vi "Load_Breast_Cancer.vi"(8 "error in":errorcluster caption="entrée d'erreur") -> (0 "error out":errorcluster caption="sortie d'erreur", 3 "Tableau":string[][](array[string]))   [LabVIEW 2020]
doc: "Data Set Characteristics :\n\nNumber of Instances : 569\n\nNumber of Attributes : 30 numeric, predictive attributes and the class\n\nAttribute Information : \n - radius (mean of distances from center to points on the perimeter)\n - texture (standard deviation of gray-scale values)\n - perimeter\n - area\n - smoothness (local variation in radius lengths)\n - compactness (perimeter^2 / area - 1.0)\n - concavity (severity of concave portions of the contour)\n - concave points (number of concave portions of the contour)\n - symmetry\n - fractal dimension (“coastline approximation” - 1)\n\nThe mean, standard error, and “worst” or largest (mean of the three worst/largest values) of these features were computed for each image, resulting in 30 features. For instance, field 0 is Mean Radius, field 10 is Radius SE, field 20 is Worst Radius.\n\nclass :\n - WDBC-Malignant\n - WDBC-Benign\n\nSummary Statistics : \n\n - radius (mean) : 6.981 28.11\n - texture (mean) : 9.71 39.28\n - perimeter (mean) : 43.79 188.5\n - area (mean) : 143.5 2501.0\n - smoothness (mean) : 0.053 0.163\n - compactness (mean) : 0.019 0.345\n - concavity (mean) : 0.0 0.427\n - concave points (mean) : 0.0 0.201\n - symmetry (mean) : 0.106 0.304\n - fractal dimension (mean) : 0.05 0.097\n - radius (standard error) : 0.112 2.873\n - texture (standard error) : 0.36 4.885\n - perimeter (standard error) : 0.757 21.98\n - area (standard error) : 6.802 542.2\n - smoothness (standard error) : 0.002 0.031\n - compactness (standard error) : 0.002 0.135\n - concavity (standard error) : 0.0 0.396\n - concave points (standard error) : 0.0 0.053\n - symmetry (standard error) : 0.008 0.079\n - fractal dimension (standard error): 0.001 0.03\n - radius (worst) : 7.93 36.04\n - texture (worst) : 12.02 49.54\n - perimeter (worst) : 50.41 251.2\n - area (worst) : 185.2 4254.0\n - smoothness (worst) : 0.071 0.223\n - compactness (worst) : 0.027 1.058\n - concavity (worst) : 0.0 1.252\n - concave points (worst) : 0.0 0.291\n - symmetry (worst) : 0.156 0.664\n - fractal dimension (worst) : 0.055 0.208\n\nMissing Attribute Values : None\n\nClass Distribution : \n - 212 - Malignant \n - 357 - Benign\n\nCreator : Dr. William H. Wolberg, W. Nick Street, Olvi L. Mangasarian\n\nDonor : Nick Street\n\nDate : November, 1995\n\nThis is a copy of UCI ML Breast Cancer Wisconsin (Diagnostic) datasets. https://goo.gl/U2Uwz2\n\nFeatures are computed from a digitized image of a fine needle aspirate (FNA) of a breast mass. They describe characteristics of the cell nuclei present in the image.\n\nSeparating plane described above was obtained using Multisurface Method-Tree (MSM-T) [K. P. Bennett, “Decision Tree Construction Via Linear Programming.” Proceedings of the 4th Midwest Artificial Intelligence and Cognitive Science Society, pp. 97-101, 1992], a classification method which uses linear programming to construct a decision tree. Relevant features were selected using an exhaustive search in the space of 1-4 features and 1-3 separating planes.\n\nThe actual linear program used to obtain the separating plane in the 3-dimensional space is that described in: [K. P. Bennett and O. L. Mangasarian: “Robust Linear Programming Discrimination of Two Linearly Inseparable Sets”, Optimization Methods and Software 1, 1992, 23-34].\n\nThis database is also available through the UW CS ftp server:\n\nftp ftp.cs.wisc.edu cd math-prog/cpo-dataset/machine-learn/WDBC/"
uses:
  Load_Breast_Cancer.lvclass
panel:
  out "Load_Breast_Cancer en sortie":refnum<class "Load_Breast_Cancer.lvclass">
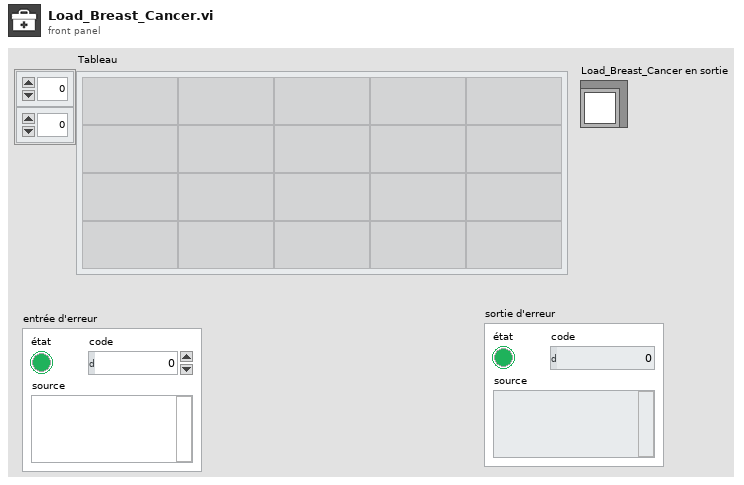
[diagram p1: front panel]
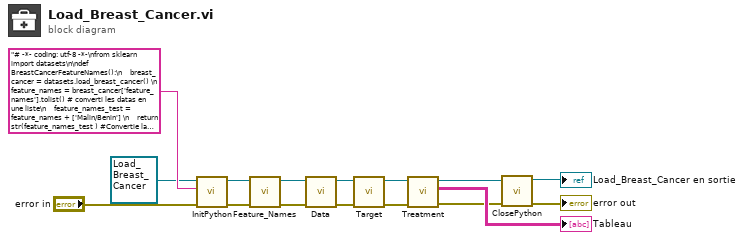
[diagram p0: block diagram]
diagram:
  n1 = call-dynamic "InitPython.vi"("error in (no error)"="error in", "Python Instruction"="# -*- coding: utf-8 -*-\nfrom sklearn import datasets\n\ndef BreastCancerFeatureNames():\n    breast_cancer = datasets.load_breast_cancer() \n    feature_names = breast_cancer['feature_names'].tolist() # converti les datas en une liste\n    feature_names_test = feature_names + ['Malin/Benin'] \n    return str(feature_names_test ) #Convertie la liste en string\n\ndef BreastCancerData():\n    breast_cancer = datasets.load_breast_cancer() \n    data = breast_cancer['data'].tolist() # converti les datas en une liste\n    return str(data) #Convertie la liste en string\n\ndef BreastCancerTarget():\n    breast_cancer = datasets.load_breast_cancer() \n    data_target = breast_cancer['target'].tolist() # converti les datas en une liste\n    return str(data_target) #Convertie la liste en string", "Scikit-learn en entrée"=refnum<class "Load_Breast_Cancer.lvclass"> refnum ("Load_Breast_Cancer.lvclass")) -> ("error out"=w11:errorcluster, "Scikit-learn en sortie"=w12:refnum<class "Load_Breast_Cancer.lvclass">)  [unwired: 7 in]
  n2 = call-dynamic "Feature_Names.vi"("error in (no error)"=w11, "Load_Breast_Cancer en entrée"=w12) -> ("error out"=w9:errorcluster, "Load_Breast_Cancer en sortie"=w10:refnum<class "Load_Breast_Cancer.lvclass">)  [unwired: 8 in]
  n3 = call-dynamic "Data.vi"("error in (no error)"=w9, "Load_Breast_Cancer en entrée"=w10) -> ("error out"=w7:errorcluster, "Load_Breast_Cancer en sortie"=w8:refnum<class "Load_Breast_Cancer.lvclass">)  [unwired: 8 in]
  n4 = call-dynamic "Target.vi"("error in (no error)"=w7, "Load_Breast_Cancer en entrée"=w8) -> ("error out"=w5:errorcluster, "Load_Breast_Cancer en sortie"=w6:refnum<class "Load_Breast_Cancer.lvclass">)  [unwired: 8 in]
  n5 = call-dynamic "Treatment.vi"("error in (no error)"=w5, "Load_Breast_Cancer en entrée"=w6) -> ("error out"=w2:errorcluster, "Tableau"=→"Tableau":string[][], "Load_Breast_Cancer en sortie"=w4:refnum<class "Load_Breast_Cancer.lvclass">)  [unwired: 7 in]
  n6 = call-dynamic "ClosePython.vi"("error in (no error)"=w2, "Scikit-learn en entrée"=w4) -> ("error out"=→"error out":errorcluster, "Scikit-learn en sortie"=→"Load_Breast_Cancer en sortie":refnum<class "Load_Breast_Cancer.lvclass">)  [unwired: 8 in]
